vi "Write Event Source Enqueuer.vi"(8 "error in (no error)":errorcluster, 10 "Source Actro:Message Enqueuer":refnum<class "Message Enqueuer.lvclass">, 11 "Event Sink in":refnum<class "Event Sink.lvclass">) -> (0 "error out":errorcluster, 3 "Event Sink out":refnum<class "Event Sink.lvclass">)   [LabVIEW 2016, in "Event Source.lvlib" / "Event Sink.lvclass"]
uses:
  Event Sink.lvclass
  <vilib>/ActorFramework/Message Enqueuer/Message Enqueuer.lvclass
  Event Sink.lvclass/Event Sink.ctl
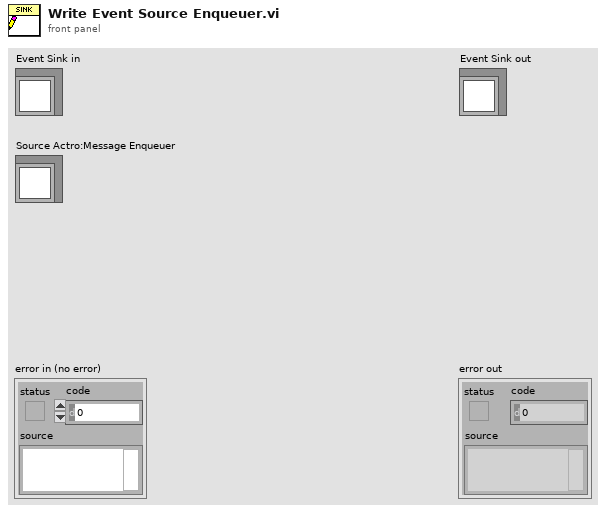
[diagram p1: front panel]
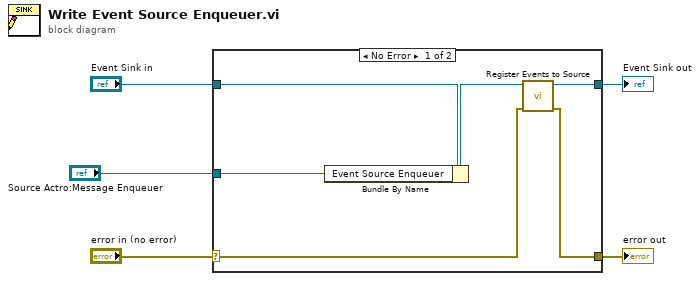
[diagram p0: block diagram]
diagram:
  n1 = case shown="No Error" "error in (no error)" {
    selector: "error in (no error)" -> [w7 w12]
    tunnel: [w6 w12] -> w4
    tunnel: [w8 w13] -> w2
    tunnel: "Event Sink in" -> [w11 w13]
    tunnel: "Source Actro:Message Enqueuer" -> [w10 _]
    frame No Error {
      n2 = Bundle By Name(cluster=w11, "Event Source Enqueuer"=w10) -> (w9:refnum<class "Event Sink.lvclass">)
      n3 = call-dynamic "Register Events to Source.vi"("error in (no error)"=w7, "Event Sink in"=w9) -> ("error out"=w6:errorcluster, "Event Sink out"=w8:refnum<class "Event Sink.lvclass">)  [unwired: 8 in]
    }
    frame Error {
    }
  }
  "error out" <- w4
  "Event Sink out" <- w2
